vi "initialize.vi"(8 "error in (no error)":errorcluster caption="错误输入（无错误）", 11 "2700 输入":refnum<class "2700.lvclass">) -> (0 "error out":errorcluster caption="错误输出", 3 "2700 输出":refnum<class "2700.lvclass">)   [LabVIEW 2021, in "2700.lvclass"]
uses:
  2700.lvclass
  DMM/DMM.lvclass
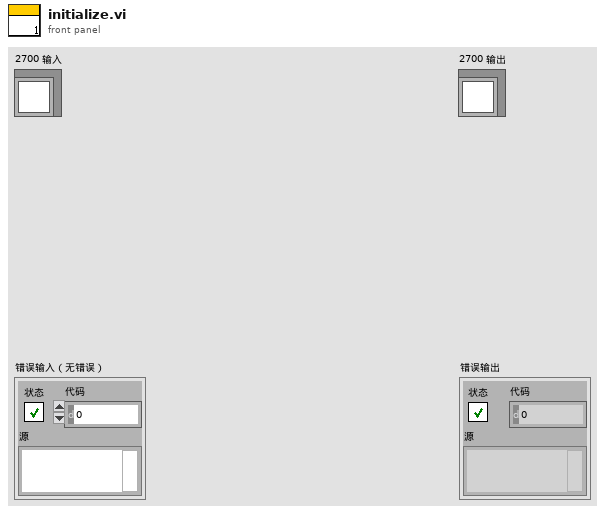
[diagram p1: front panel]
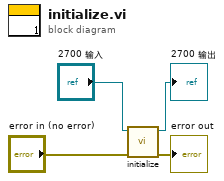
[diagram p0: block diagram]
diagram:
  n1 = call-parent "initialize.vi"("error in (no error)"="error in (no error)", "DMM 输入"="2700 输入") -> ("error out"=→"error out":errorcluster, "DMM 输出"=→"2700 输出":refnum<class "2700.lvclass">)  [unwired: 8 in]
